vi "RvsTime_Tektronix_Vbias_crh.vi"() -> ()   [LabVIEW 2017]
uses:
  sub_vis/ke26xx/Public/Channel.ctl
  sub_vis/ke26xx/KE26XX.lvlib
panel:
  out "Total filename":string="C:\\THz-Data\\Vacuum_Box\\110725"
  in  "Heater Range (0: Off)":u16(ring) items=["Off", "Low (0.5W)", "Med (5W)", "High (50W)"]
  in  "Plot Options":enum32{"dI/dV vs V", "I vs V", "Temperature"}(tab)
  out "G vs V at neg times":cluster{"Y":dbl[], "Y":dbl[]}[](graph)
  out "G vs V at max. response":cluster{"Y":dbl[], "Y":dbl[]}[](graph)
  out "I vs V at neg times":cluster{"Y":dbl[], "Y":dbl[]}[](graph)
  out "I vs V at max. response":cluster{"Y":dbl[], "Y":dbl[]}[](graph)
  out "temp vs time":cluster{"Y":dbl[], "Y":dbl[]}[](graph)
  in  "Device Control":T1(tab)=enum."Record Data"
  in  "Lakeshore Input (0: A)":u16(ring)=2 items=["A", "B", "ITC5035"]
  in  "Lakeshore VISA Session":refnum<visa-resource-name>="COM1"
  in  "Log Temp":bool=TRUE
  in  "Heater Control":enum32{"Configure", "Heater", "Set Point"}(tab)
  in  "Curve Number (0)":dbl min=0.0 max=41.0 step=1.0
  in  "Sensor Type (0: Silicon Diode)":i8(ring) items=["Silicon Diode", "GaAIAS Diode", "100 Ohm Platinum/250", "100 Ohm Platinum/500", "1000 Ohm Platinum", "NTC RTD", "Thermo/25mV", "Thermo/50mV"]
  in  "Manual Output (%)":dbl min=0.0 max=100.0 step=0.001 format="%.;%.3f"
  in  "Loop (0: 1)":u16(ring) items=["1", "2"]
  out "Heater Output":dbl(slide) scale=0.0..100.0
  in  "Rate (D)":dbl min=0.0 max=1000.0 step=0.1 format="%.;%.1f"
  in  "Reset (I)":dbl min=0.0 max=1000.0 step=0.1 format="%.;%.1f"
  in  "Gain (P)":dbl min=0.0 max=1000.0 step=0.1 format="%.;%.1f"
  in  "Control Mode (0: Manual PID)":u16(ring) items=["Manual PID", "Zone", "Open Loop", "AutoTune PID", "AutoTune PI", "AutoTune P"]
  in  "Ramp Rate\n(K/min)":dbl=0.1 min=0.0 max=100.0 step=0.1 format="%.1f"
  in  "Ramping \nOn/Off (F: Off)":bool
  in  "Setpoint (K)":dbl min=0.0 max=1000.0 step=0.1 format="%.;%.1f"
  in  "Update":bool caption="Boolean"
  in  "Control Temp":bool=TRUE
  in  "Apply Bias":bool
  in  "Keithley VISA Session":refnum<visa-resource-name>
  in  "Channel (A):":T2
  in  "Limit (mA)":dbl=1.0 format="%.;%#_g"
  in  "Level (mV)":dbl=1.0 format="%.;%#_g"
  in  "Tektronix VISA Session":refnum<visa-resource-name>
  in  "Channel:":u16(ring) items=["Channel 1", "Channel 2", "Channel 3", "Channel 4"]
  in  "Read Scope":bool
  in  "Max. Bias (mV)":dbl=1.0 format="%.;%#_g"
  in  "Step Size (mV)":dbl=1.0 format="%.;%#_g"
  in  "Step Bias":bool
  out "Current Bias (mV)":dbl=1.0 format="%.;%#_g"
  out "Node":string
  in  "Stop 2":bool
  in  "Path":string="C:\\path\\to\\file"
  in  "Filename":string="filename"
  in  "Extension":string=".dat"
  in  "Comments":string="comments"
  in  "Start":bool
  in  "Number of Scans:":i32
  in  "Plot Scales":u16(ring) items=["Autoscale All", "Autoscale X", "Autoscale Y", "Manual Scale"]
  out "Current (mA):":dbl=19.983 format="%.;%.4f"
  out "Voltage (mV):":dbl=19.983 format="%.;%.4f"
  in  "Y Max.":dbl min=0.0 max=1000.0 step=0.1 format="%.;%.1f"
  in  "Y Min.":dbl min=0.0 max=1000.0 step=0.1 format="%.;%.1f"
  in  "X Max.":dbl min=0.0 max=1000.0 step=0.1 format="%.;%.1f"
  in  "X Min.":dbl min=0.0 max=1000.0 step=0.1 format="%.;%.1f"
  in  "Reset":bool
  out "Resistance (Ohms)":dbl=19.983 format="%.;%_5f"
  in  "Filename 2":string="07_YBCO_EOS_20K_outofplane_pumpon_5ps_"
  out "Temperature (K)":dbl=19.983 format="%.2f"
  in  "Stop":bool
  out "Osci Readout":cluster{"Y":dbl[], "Y":dbl[]}[](graph)
  # "Temperature Sensor"
  # "Heater Control"
  # "Source Meter"
  # "Oscilloscope"
  # "Set Filename and Path"
  # "(Only when not ramping bias.)"
  # "Written by Cassi Hunt, January 2013\n\nTemperature Control: LakeShore 331\nSourceMeter: Keithley 2635A\nOscilloscope: Tektronix 7xxx Series"
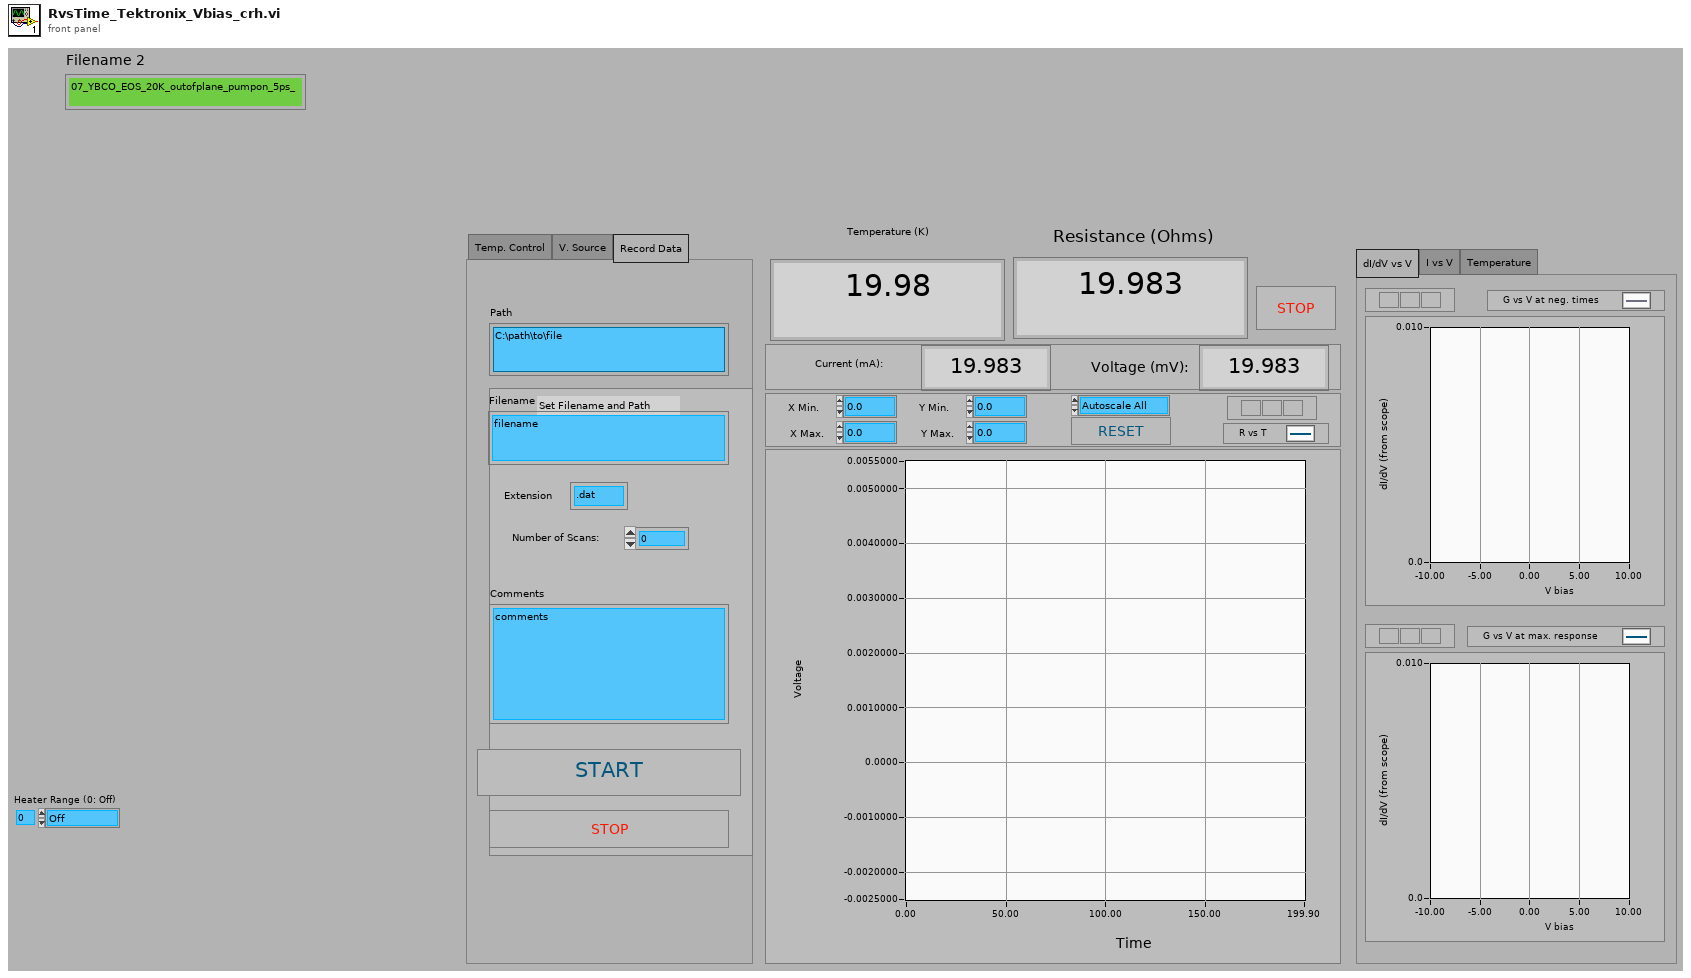
[diagram p1: front panel]
types:
  T1 = enum32{"Temp. Control", "V. Source", "Record Data"}
  T2 = typedef "KE26XX.lvlib/Channel.ctl" = enum32{"Channel A", "Channel B"}
  T3 = enum32{"Current", "Voltage", "IV", "Resistance", "Power"}
  T4 = typedef "ke26xx.lvlib/Channel.ctl" = enum32{"Channel A", "Channel B"}
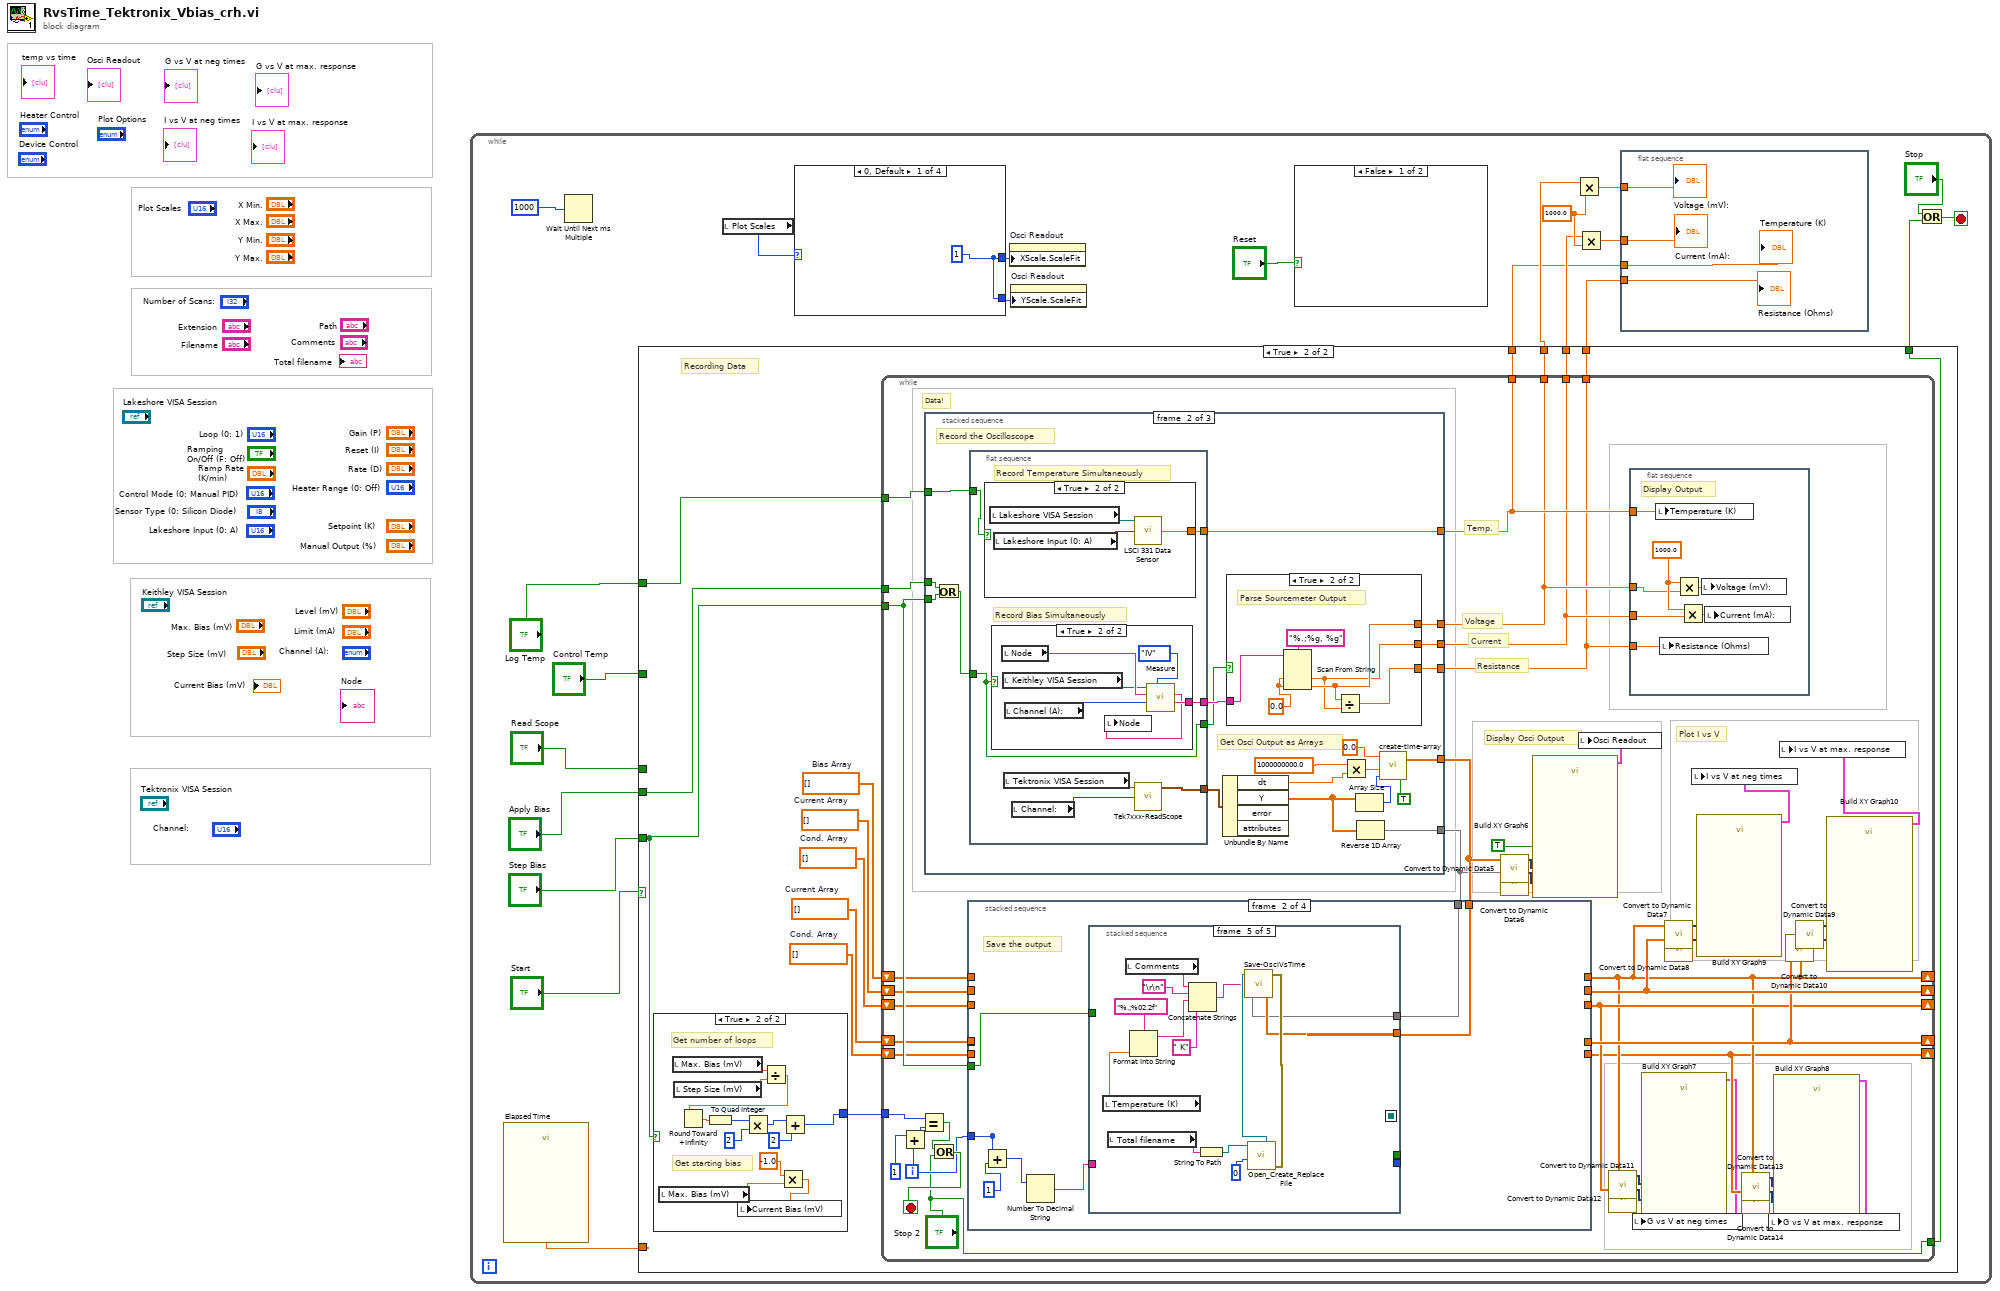
[diagram p0: block diagram]
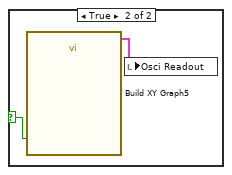
[diagram p2: hidden frame]
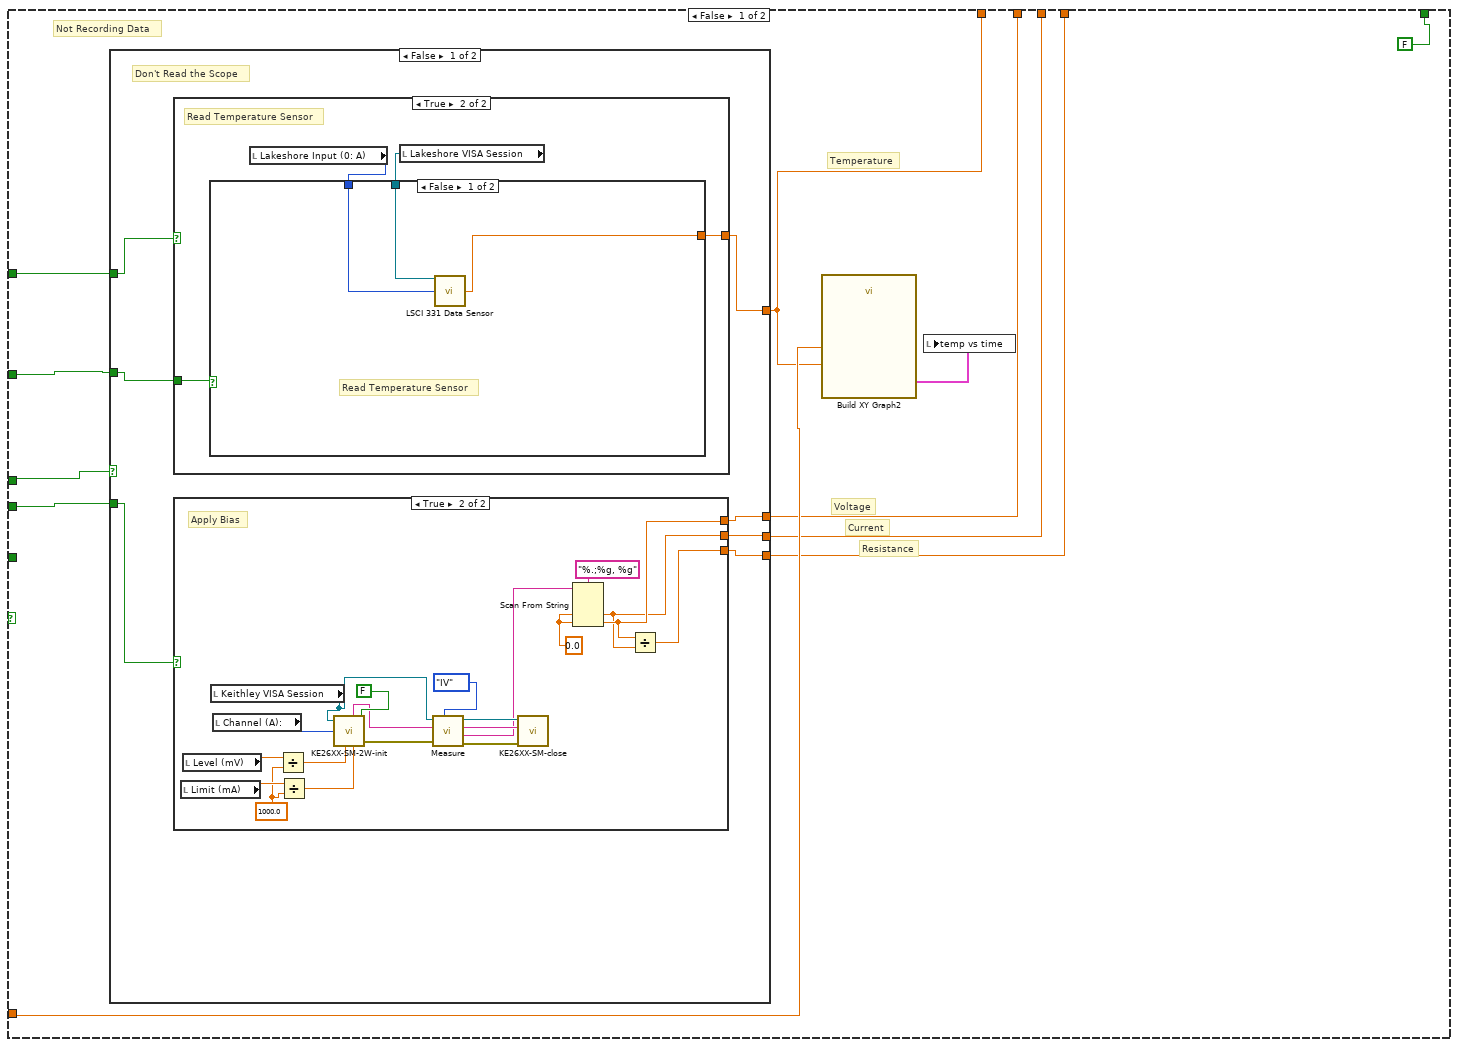
[diagram p3: hidden frame]
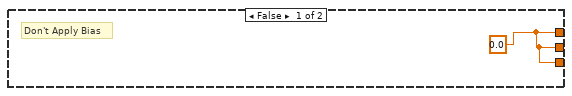
[diagram p4: hidden frame]
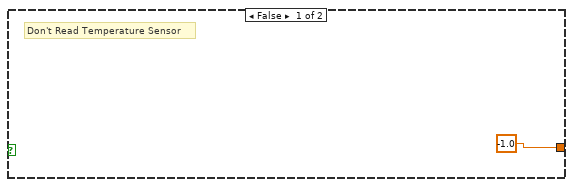
[diagram p5: hidden frame]
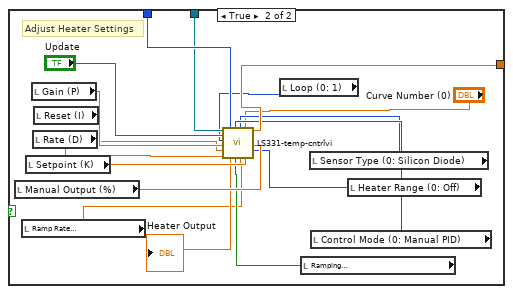
[diagram p6: hidden frame]
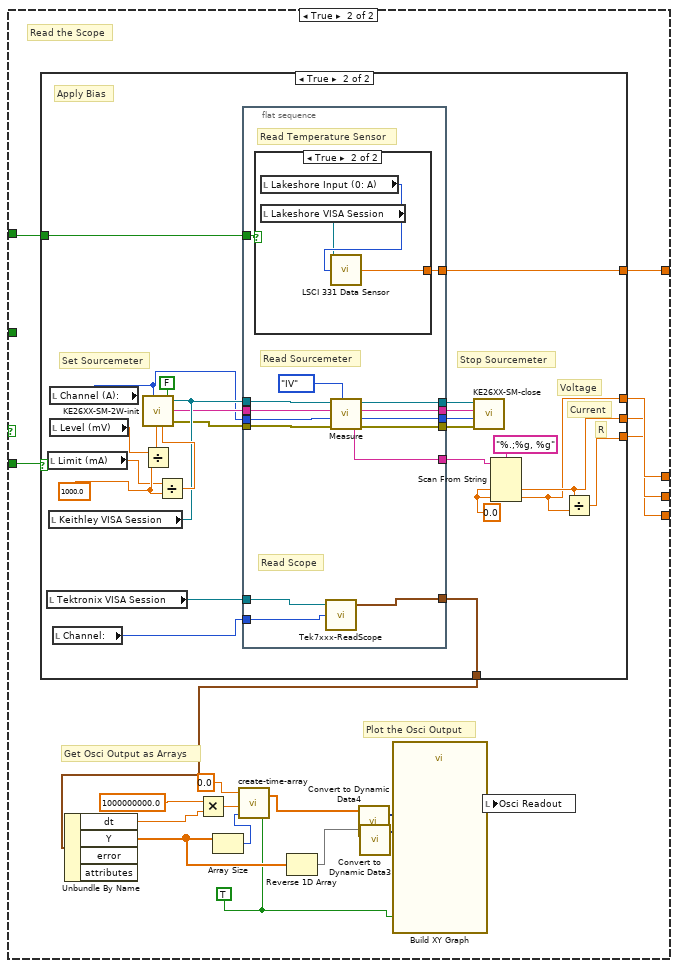
[diagram p7: hidden frame]
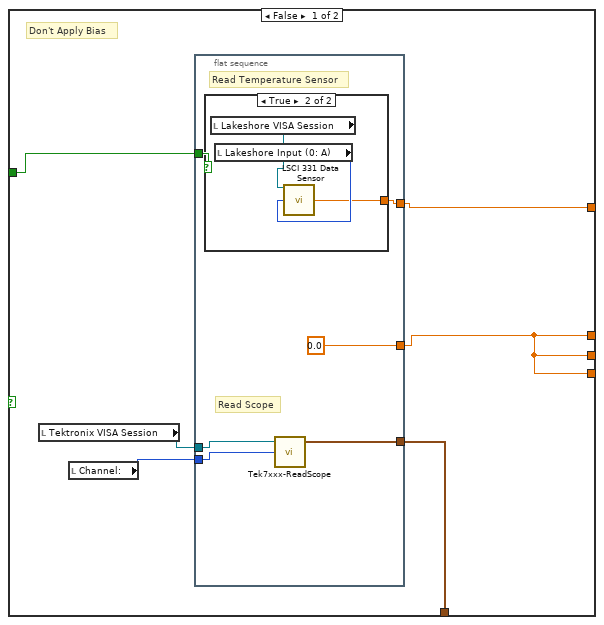
[diagram p8: hidden frame]
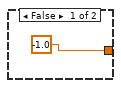
[diagram p9: hidden frame]
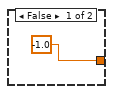
[diagram p10: hidden frame]
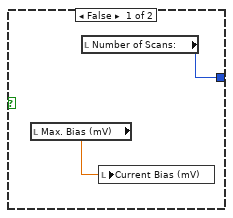
[diagram p11: hidden frame]
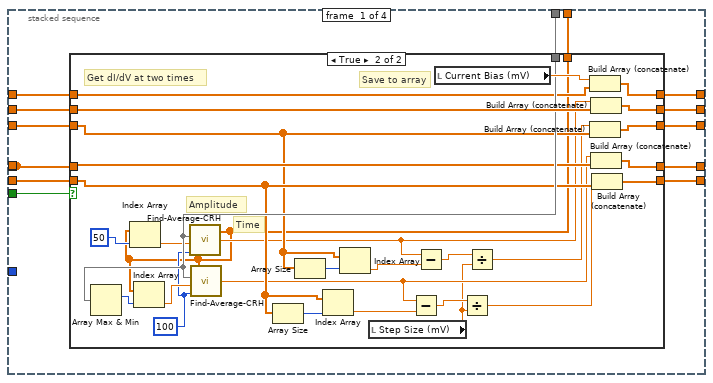
[diagram p12: hidden frame]
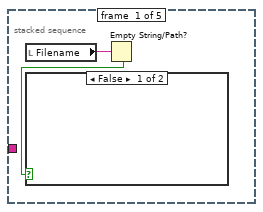
[diagram p14: hidden frame]
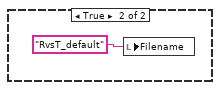
[diagram p15: hidden frame]
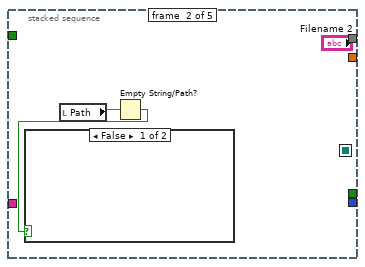
[diagram p16: hidden frame]
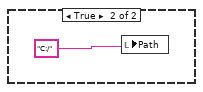
[diagram p17: hidden frame]
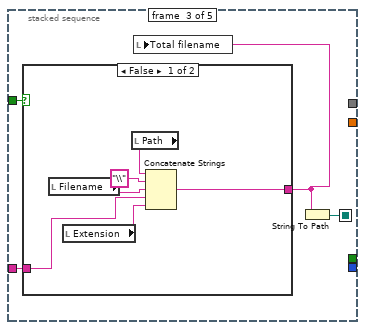
[diagram p18: hidden frame]
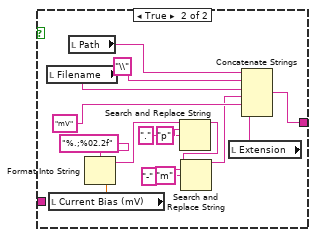
[diagram p19: hidden frame]
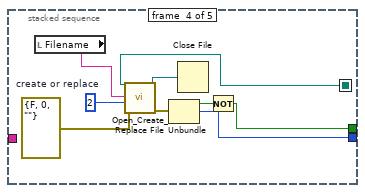
[diagram p20: hidden frame]
diagram:
  n1 = while {
    stop <- w3 stop-if-true
    w12 = 1000.0
    n2 = call "Elapsed Time"() -> ("Elapsed Time (s)"=w17:dbl)  [unwired: 12 in, 7 out]
    n3 = Wait Until Next ms Multiple(millisecond multiple=u32 1000) -> ()  [unwired: 1 out]
    n4 = case shown="True" "Start" {
      tunnel: w17 -> [w39 _]
      tunnel: "Apply Bias" -> [w35 w182]
      tunnel: [FALSE w173] -> w1
      tunnel: "Read Scope" -> [w37 _]
      tunnel: "Log Temp" -> [w36 w183]
      tunnel: "Control Temp" -> [w34 _]
      tunnel: [w33 w179] -> w9
      tunnel: [w32 w178] -> w8
      tunnel: [w31 w177] -> w7
      tunnel: [w30 w180] -> w6
      tunnel: "Step Bias" -> [_ w181]
      frame False {
        # "Temperature"
        # "Resistance"
        # "Current"
        # "Voltage"
        # "Not Recording Data"
        n5 = case shown="False" w37 {
          tunnel: w36 -> [w45 w111]
          tunnel: w35 -> [w43 w110]
          tunnel: [w44 w96] -> w30
          tunnel: w34 -> [w46 _]
          tunnel: [w42 w95] -> w33
          tunnel: [w41 w94] -> w32
          tunnel: [w40 w93] -> w31
          frame False {
            # "Don't Read the Scope"
            n6 = case shown="True" w45 {
              tunnel: [-1.0 w71] -> w44
              tunnel: w46 -> [_ w72]
              frame False {
                # "Don't Read Temperature Sensor"
              }
              frame True {
                # "Read Temperature Sensor"
                n7 = local read "Lakeshore Input (0: A)"() -> (w69:u16)
                n8 = local read "Lakeshore VISA Session"() -> (w70:refnum<visa-resource-name>)
                n9 = case shown="False" w72 {
                  tunnel: w69 -> [w74 w92]
                  tunnel: w70 -> [w75 w91]
                  tunnel: [w73 w83] -> w71
                  frame False {
                    # "Read Temperature Sensor"
                    n10 = call "LSCI 331 Data Sensor.vi"("VISA session"=w75, "Input (0: A)"=w74) -> ("Kelvin Reading"=w73:dbl)  [unwired: 1 in, 12 out]
                  }
                  frame True {
                    # "Adjust Heater Settings"
                    n11 = local read "Manual Output (%)"() -> (w85:dbl)
                    n12 = local read "Ramp Rate\n(K/min)"() -> (w80:dbl)
                    n13 = local read "Setpoint (K)"() -> (w86:dbl)
                    n14 = local read "Gain (P)"() -> (w89:dbl)
                    n15 = local read "Rate (D)"() -> (w87:dbl)
                    n16 = local read "Reset (I)"() -> (w88:dbl)
                    n17 = local read "Loop (0: 1)"() -> (w81:u16)
                    n18 = local read "Ramping \nOn/Off (F: Off)"() -> (w82:bool)
                    n19 = local read "Sensor Type (0: Silicon Diode)"() -> (w77:i8)
                    n20 = local read "Control Mode (0: Manual PID)"() -> (w78:u16)
                    n21 = local read "Heater Range (0: Off)"() -> (w79:u16)
                    n22 = call "LS331-temp-cntrlvi.vi"("VISA resource name"=w91, "Configure (False)"="Update", "Loop (0: 1)"=w81, "Gain (P) (0.0)"=w89, "Reset (I) (0.0)"=w88, "Rate (D) (0)"=w87, "Input (0: A)"=w92, "Control Mode (0: Manual PID)"=w78, "Ramping On/Off (F: Off)"=w82, "Sensor Type (0: Silicon Diode)"=w77, "Rate Value (0.1)"=w80, "Curve Number (0)"="Curve Number (0)", "Setpoint (0.0000)"=w86, "Manual Output (0.000)"=w85, "Heater Range (0: Off)"=w79) -> ("Loop 1\nHeater Output"=→"Heater Output":dbl, "Kelvin Reading"=w83:dbl)  [unwired: 1 in, 2 out]
                  }
                }
              }
            }
            n23 = case shown="True" w43 {
              tunnel: [w47 w49] -> w42
              tunnel: [w47 w48] -> w41
              tunnel: [w47 w51] -> w40
              frame False {
                w47 = 0.0
                # "Don't Apply Bias"
              }
              frame True {
                w53 = 0.0
                w63 = 1000.0
                # "Apply Bias"
                n24 = local read "Limit (mA)"() -> (w65:dbl)
                n25 = local read "Level (mV)"() -> (w67:dbl)
                n26 = local read "Keithley VISA Session"() -> (w59:refnum<visa-resource-name>)
                n27 = local read "Channel (A):"() -> (w62:T4)
                n28 = Divide(x=w67, y=w63) -> (x/y=w66:dbl)
                n29 = Divide(x=w65, y=w63) -> (x/y=w64:dbl)
                n30 = call "KE26XX-SM-2W-init.vi"("VISA resource name"=w59, "Channel (Channel A)"=w62, "Level"=w66, "Error Query (False)"=FALSE, "Limit"=w64) -> ("Node Out"=w60:string, "error out"=w58:errorcluster)  [unwired: 3 in]
                n31 = call "Measure.vi"("Function (Current)"=T3."IV" ("Measure Function (Current)"), "error in (no error)"=w58, "Node In"=w60, "VISA resource name"=w59) -> ("error out"=w54:errorcluster, "Output"=w50:string, "Node Out"=w56:string, "VISA resource name out"=w55:refnum<visa-resource-name>)  [unwired: 3 in, 1 out]
                n32 = call "KE26XX-SM-close.vi"("error in (no error)"=w54, "Node In"=w56, "VISA resource name"=w55) -> ()  [unwired: 8 in, 1 out]
                n33 = Scan From String(format string="%.;%g, %g", input string=w50, default 1=w53, default 2=w53) -> (output 1=w48:dbl, output 2=w49:dbl)  [unwired: 2 in, 3 out]
                n34 = Divide(x=w49, y=w48) -> (x/y=w51:dbl)
              }
            }
          }
          frame True {
            w100 = TRUE
            # "Plot the Osci Output"
            # "Get Osci Output as Arrays"
            # "Read the Scope"
            n35 = case shown="True" w110 {
              tunnel: w111 -> [w117 w152]
              tunnel: [w115 w128] -> w95
              tunnel: [w115 w129] -> w94
              tunnel: [w115 w134] -> w93
              tunnel: [w116 w131] -> w96
              tunnel: [w112 w130] -> w99
              frame False {
                # "Don't Apply Bias"
                n36 = local read "Tektronix VISA Session"() -> (w114:refnum<visa-resource-name>)
                n37 = local read "Channel:"() -> (w113:u16)
                n38 = flat-sequence {
                  tunnel: w117 -> [w123]
                  tunnel: [w122] -> w116
                  tunnel: [0.0] -> w115
                  tunnel: w114 -> [w120]
                  tunnel: w113 -> [w119]
                  tunnel: [w118] -> w112
                  frame #0 {
                    # "Read Scope"
                    # "Read Temperature Sensor"
                    n39 = case shown="True" w123 {
                      tunnel: [-1.0 w125] -> w122
                      frame False {
                      }
                      frame True {
                        n40 = local read "Lakeshore VISA Session"() -> (w127:refnum<visa-resource-name>)
                        n41 = local read "Lakeshore Input (0: A)"() -> (w126:u16)
                        n42 = call "LSCI 331 Data Sensor.vi"("VISA session"=w127, "Input (0: A)"=w126) -> ("Kelvin Reading"=w125:dbl)  [unwired: 1 in, 12 out]
                      }
                    }
                    n43 = call "Tek7xxx-ReadScope.vi"("Channel (0: Channel 1)"=w119, "VISA Resource Name"=w120) -> ("Waveform Graph"=w118:waveform(dbl))  [unwired: 3 in]
                  }
                }
              }
              frame True {
                w137 = 0.0
                w151 = 1000.0
                # "R"
                # "Current"
                # "Voltage"
                # "Stop Sourcemeter"
                # "Set Sourcemeter"
                # "Apply Bias"
                n44 = local read "Tektronix VISA Session"() -> (w133:refnum<visa-resource-name>)
                n45 = local read "Limit (mA)"() -> (w148:dbl)
                n46 = local read "Keithley VISA Session"() -> (w145:refnum<visa-resource-name>)
                n47 = local read "Channel (A):"() -> (w142:T4)
                n48 = local read "Level (mV)"() -> (w147:dbl)
                n49 = local read "Channel:"() -> (w132:u16)
                n50 = Divide(x=w147, y=w151) -> (x/y=w149:dbl)
                n51 = Divide(x=w148, y=w151) -> (x/y=w150:dbl)
                n52 = call "KE26XX-SM-2W-init.vi"("VISA resource name"=w145, "Channel (Channel A)"=w142, "Level"=w149, "Error Query (False)"=FALSE, "Limit"=w150) -> ("Node Out"=w144:string, "error out"=w143:errorcluster)  [unwired: 3 in]
                n53 = flat-sequence {
                  tunnel: [w166] -> w131
                  tunnel: w152 -> [w165]
                  tunnel: w144 -> [w164]
                  tunnel: w145 -> [w163]
                  tunnel: w143 -> [w162]
                  tunnel: w142 -> [w157]
                  tunnel: [w161] -> w139
                  tunnel: [w160] -> w135
                  tunnel: [w159] -> w140
                  tunnel: [w158] -> w141
                  tunnel: [w157] -> w138
                  tunnel: w133 -> [w156]
                  tunnel: w132 -> [w155]
                  tunnel: [w154] -> w130
                  frame #0 {
                    # "Read Scope"
                    # "Read Sourcemeter"
                    # "Read Temperature Sensor"
                    n54 = case shown="True" w165 {
                      tunnel: [-1.0 w168] -> w166
                      frame False {
                      }
                      frame True {
                        n55 = local read "Lakeshore Input (0: A)"() -> (w170:u16)
                        n56 = local read "Lakeshore VISA Session"() -> (w169:refnum<visa-resource-name>)
                        n57 = call "LSCI 331 Data Sensor.vi"("VISA session"=w169, "Input (0: A)"=w170) -> ("Kelvin Reading"=w168:dbl)  [unwired: 1 in, 12 out]
                      }
                    }
                    n58 = call "Tek7xxx-ReadScope.vi"("Channel (0: Channel 1)"=w155, "VISA Resource Name"=w156) -> ("Waveform Graph"=w154:waveform(dbl))  [unwired: 3 in]
                    n59 = call "Measure.vi"("Function (Current)"=T3."IV" ("Measure Function (Current)"), "error in (no error)"=w162, "Channel (Channel A)"=w157, "Node In"=w164, "VISA resource name"=w163) -> ("error out"=w161:errorcluster, "Output"=w160:string, "Node Out"=w159:string, "VISA resource name out"=w158:refnum<visa-resource-name>)  [unwired: 2 in, 1 out]
                  }
                }
                n60 = call "KE26XX-SM-close.vi"("error in (no error)"=w139, "Channel (Channel A)"=w138, "Node In"=w140, "VISA resource name"=w141) -> ()  [unwired: 7 in, 1 out]
                n61 = Scan From String(format string="%.;%g, %g", input string=w135, default 1=w137, default 2=w137) -> (output 1=w129:dbl, output 2=w128:dbl)  [unwired: 2 in, 3 out]
                n62 = Divide(x=w129, y=w128) -> (x/y=w134:dbl)
              }
            }
            n63 = Unbundle By Name(w99) -> ("dt"=w105:dbl, "Y"=w104:dbl[])  [unwired: 2 out]
            n64 = Multiply(x=1000000000.0, y=w105) -> (x*y=w107:dbl)
            n65 = Array Size(array=w104) -> (size(s)=w109:i32)
            n66 = call "create-time-array.vi"("Invert"=w100, "Array Size"=w109, "dt"=w107, "t0"=0.0) -> ("Time Array"=w98:dbl[])
            n67 = Reverse 1D Array(array=w104) -> (reversed array=w97:dbl[])
            n68 = call "Convert to Dynamic Data4"("Array"=w98) -> ("Dynamic Data Type"=w103:dynamicdata)  [unwired: 3 in]
            n69 = call "Convert to Dynamic Data3"("Array"=w97) -> ("Dynamic Data Type"=w102:dynamicdata)  [unwired: 3 in]
            n70 = call "Build XY Graph"("Reset"=w100, "Y Input"=w102, "X Input"=w103) -> ("XY Graph"=w101:cluster{"Y":dbl[], "Y":dbl[]}[])  [unwired: 2 in, 6 out]
            n71 = local write "Osci Readout"(w101) -> ()
          }
        }
        n72 = call "Build XY Graph2"("Y Input"=w30, "X Input"=w39) -> ("XY Graph"=w38:cluster{"Y":dbl[], "Y":dbl[]}[])  [unwired: 3 in, 6 out]
        n73 = local write "temp vs time"(w38) -> ()
      }
      frame True {
        w171 = dbl[] []  # Cond. Array
        w172 = dbl[] []  # Current Array
        w174 = dbl[] []  # Cond. Array
        w175 = dbl[] []  # Current Array
        w176 = dbl[] []  # Bias Array
        # "Recording Data"
        n74 = case shown="True" w181 {
          tunnel: [w185 w190] -> w184
          frame False {
            n75 = local read "Max. Bias (mV)"() -> (w186:dbl)
            n76 = local read "Number of Scans:"() -> (w185:i32)
            n77 = local write "Current Bias (mV)"(w186) -> ()
          }
          frame True {
            # "Get starting bias"
            # "Get number of loops"
            n78 = local read "Max. Bias (mV)"() -> (w188:dbl)
            n79 = local read "Max. Bias (mV)"() -> (w198:dbl)
            n80 = local read "Step Size (mV)"() -> (w197:dbl)
            n81 = Divide(x=w198, y=w197) -> (x/y=w196:dbl)
            n82 = Round Toward +Infinity(x=w196) -> (ceil(x): smallest int >= x=w193:dbl)
            n83 = To Quad Integer(1:w193) -> (0:w192:i64)
            n84 = Multiply(x=w192, y=2) -> (x*y=w194:i64)
            n85 = Multiply(x=-1.0, y=w188) -> (x*y=w187:dbl)
            n86 = local write "Current Bias (mV)"(w187) -> ()
            n87 = Add(x=w194, y=2) -> (x+y=w190:i64)
          }
        }
        n88 = while {
          tunnel: w184 -> [w240]
          tunnel: w183 -> [w239]
          tunnel: w182 -> [w238]
          tunnel: w181 -> [w227]
          tunnel: [w237] -> w180
          tunnel: [w236] -> w179
          tunnel: [w235] -> w178
          tunnel: [w234] -> w177
          shift-right: [w210] -> _
          shift-left: w176 -> [w226]
          shift-right: [w218] -> _
          shift-left: w175 -> [w225]
          shift-right: [w212] -> _
          shift-left: w174 -> [w224]
          tunnel: ["Stop 2"] -> w173
          shift-right: [w215] -> _
          shift-left: w172 -> [w221]
          shift-right: [w208] -> _
          shift-left: w171 -> [w220]
          i -> [w202]
          stop <- w222 stop-if-true
          # "Plot I vs V"
          # "Display Osci Output"
          # "Resistance"
          # "Current"
          # "Voltage"
          # "Temp."
          # "Data!"
          n89 = Add(x=1, y=w202) -> (x+y=w200:i32)
          n90 = Equal?(x=w240, y=w200) -> (x = y?=w223:bool)
          n91 = stacked-sequence {
            tunnel: w239 -> [_ w389 _]
            tunnel: [_ w388 _] -> w237
            tunnel: w238 -> [w367 w385 w424]
            tunnel: w227 -> [w366 w384 w422]
            tunnel: [_ w387 _] -> w228
            tunnel: [_ w386 _] -> w229
            tunnel: [_ w380 _] -> w236
            tunnel: [_ w379 _] -> w235
            tunnel: [_ w378 _] -> w234
            frame #0 {
              n92 = Or(x=w367, y=w366) -> (x .or. y?=w368:bool)
              n93 = case shown="True" w368 {
                frame False {
                }
                frame True {
                  w375 = 1000.0
                  # "Apply Bias"
                  n94 = local read "Keithley VISA Session"() -> (w371:refnum<visa-resource-name>)
                  n95 = local read "Current Bias (mV)"() -> (w377:dbl)
                  n96 = local read "Channel (A):"() -> (w370:T4)
                  n97 = local read "Limit (mA)"() -> (w376:dbl)
                  n98 = Divide(x=w377, y=w375) -> (x/y=w374:dbl)
                  n99 = Divide(x=w376, y=w375) -> (x/y=w373:dbl)
                  n100 = call "KE26XX-SM-2W-init.vi"("VISA resource name"=w371, "Channel (Channel A)"=w370, "Level"=w374, "Error Query (False)"=FALSE, "Limit"=w373) -> ("Node Out"=w369:string)  [unwired: 3 in, 1 out]
                  n101 = local write "Node"(w369) -> ()
                }
              }
            }
            frame #1 {
              # "Get Osci Output as Arrays"
              # "Record the Oscilloscope"
              n102 = Or(x=w385, y=w384) -> (x .or. y?=w383:bool)
              n103 = flat-sequence {
                tunnel: w389 -> [w411]
                tunnel: [w410] -> w388
                tunnel: [w407] -> w397
                tunnel: w383 -> [w405]
                tunnel: [w406] -> w382
                tunnel: [w405] -> w381
                frame #0 {
                  # "Record Bias Simultaneously"
                  # "Record Temperature Simultaneously"
                  n104 = case shown="True" w411 {
                    tunnel: [-1.0 w419] -> w410
                    frame False {
                    }
                    frame True {
                      n105 = local read "Lakeshore VISA Session"() -> (w421:refnum<visa-resource-name>)
                      n106 = local read "Lakeshore Input (0: A)"() -> (w420:u16)
                      n107 = call "LSCI 331 Data Sensor.vi"("VISA session"=w421, "Input (0: A)"=w420) -> ("Kelvin Reading"=w419:dbl)  [unwired: 1 in, 12 out]
                    }
                  }
                  n108 = case shown="True" w405 {
                    tunnel: [_ w413] -> w406
                    frame False {
                    }
                    frame True {
                      n109 = local read "Node"() -> (w416:string)
                      n110 = local read "Keithley VISA Session"() -> (w415:refnum<visa-resource-name>)
                      n111 = local read "Channel (A):"() -> (w414:T4)
                      n112 = call "Measure.vi"("Function (Current)"=T3."IV" ("Measure Function (Current)"), "Channel (Channel A)"=w414, "Node In"=w416, "VISA resource name"=w415) -> ("Output"=w413:string, "Node Out"=w412:string)  [unwired: 3 in, 3 out]
                      n113 = local write "Node"(w412) -> ()
                    }
                  }
                  n114 = local read "Tektronix VISA Session"() -> (w409:refnum<visa-resource-name>)
                  n115 = local read "Channel:"() -> (w408:u16)
                  n116 = call "Tek7xxx-ReadScope.vi"("Channel (0: Channel 1)"=w408, "VISA Resource Name"=w409) -> ("Waveform Graph"=w407:waveform(dbl))  [unwired: 3 in]
                }
              }
              n117 = Unbundle By Name(w397) -> ("dt"=w394:dbl, "Y"=w395:dbl[])  [unwired: 2 out]
              n118 = case shown="True" w381 {
                tunnel: w382 -> [_ w402]
                tunnel: [w398 w400] -> w380
                tunnel: [w398 w399] -> w379
                tunnel: [w398 w403] -> w378
                frame False {
                  w398 = 0.0
                }
                frame True {
                  w401 = 0.0
                  # "Parse Sourcemeter Output"
                  n119 = Scan From String(format string="%.;%g, %g", input string=w402, default 1=w401, default 2=w401) -> (output 1=w399:dbl, output 2=w400:dbl)  [unwired: 2 in, 3 out]
                  n120 = Divide(x=w400, y=w399) -> (x/y=w403:dbl)
                }
              }
              n121 = Multiply(x=1000000000.0, y=w394) -> (x*y=w392:dbl)
              n122 = Array Size(array=w395) -> (size(s)=w390:i32)
              n123 = Reverse 1D Array(array=w395) -> (reversed array=w387:dbl[])
              n124 = call "create-time-array.vi"("Invert"=TRUE, "Array Size"=w390, "dt"=w392, "t0"=0.0) -> ("Time Array"=w386:dbl[])
            }
            frame #2 {
              n125 = Or(x=w424, y=w422) -> (x .or. y?=w423:bool)
              n126 = case shown="True" w423 {
                frame False {
                }
                frame True {
                  # "Stop Sourcemeter"
                  n127 = local read "Keithley VISA Session"() -> (w427:refnum<visa-resource-name>)
                  n128 = local read "Channel (A):"() -> (w425:T4)
                  n129 = local read "Node"() -> (w426:string)
                  n130 = call "KE26XX-SM-close.vi"("Channel (Channel A)"=w425, "Node In"=w426, "VISA resource name"=w427) -> ()  [unwired: 8 in, 1 out]
                }
              }
            }
          }
          n131 = Or(x=w223, y="Stop 2") -> (x .or. y?=w222:bool)
          n132 = stacked-sequence {
            tunnel: w229 -> [w251 w289 _ _]
            tunnel: w228 -> [w252 w290 _ _]
            tunnel: w227 -> [w253 w288 w349 _]
            tunnel: w226 -> [w250 _ _ _]
            tunnel: w225 -> [w249 _ _ _]
            tunnel: w224 -> [w248 _ _ _]
            tunnel: [w247 _ _ _] -> w210
            tunnel: [w246 _ _ _] -> w218
            tunnel: [w245 _ _ _] -> w212
            tunnel: [w244 _ _ _] -> _
            tunnel: w221 -> [w244 _ _ _]
            tunnel: [w243 _ _ _] -> w215
            tunnel: w220 -> [w242 _ _ _]
            tunnel: [w241 _ _ _] -> w208
            tunnel: [_ w293 _ _] -> _
            tunnel: w202 -> [_ w293 _ _]
            frame #0 {
              n133 = case shown="True" w253 {
                tunnel: w252 -> [_ w282]
                tunnel: w251 -> [_ w259]
                tunnel: w250 -> [w258 w262]
                tunnel: w249 -> [w257 w287]
                tunnel: w248 -> [w256 w272]
                tunnel: [w258 w286] -> w247
                tunnel: [w257 w285] -> w246
                tunnel: [w256 w284] -> w245
                tunnel: w244 -> [w255 w278]
                tunnel: [w255 w277] -> w243
                tunnel: [w254 w276] -> w241
                tunnel: w242 -> [w254 w273]
                frame False {
                }
                frame True {
                  w279 = 100
                  # "Time"
                  # "Amplitude"
                  # "Save to array"
                  # "Get dI/dV at two times"
                  n134 = Array Max & Min(array=w282) -> (max index (indices)=w281:i32)  [unwired: 3 out]
                  n135 = Index Array(array=w259, index=50) -> (element=w260:dbl)
                  n136 = Index Array(array=w259, index=w281) -> (element=w280:dbl)
                  n137 = call "Find-Average-CRH.vi"("Number to average"=w279, "t0"=w260, "Amplitude Array"=w282, "Time Array"=w259) -> ("Averaged Amplitude"=w271:dbl)
                  n138 = call "Find-Average-CRH.vi"("Number to average"=w279, "t0"=w280, "Amplitude Array"=w282, "Time Array"=w259) -> ("Averaged Amplitude"=w268:dbl)
                  n139 = Array Size(array=w273) -> (size(s)=w274:i32)
                  n140 = Array Size(array=w272) -> (size(s)=w275:i32)
                  n141 = Index Array(array=w273, index=w274) -> (element=w267:dbl)
                  n142 = Index Array(array=w272, index=w275) -> (element=w270:dbl)
                  n143 = local read "Step Size (mV)"() -> (w265:dbl)
                  n144 = Subtract(x=w268, y=w267) -> (x-y=w266:dbl)
                  n145 = Subtract(x=w271, y=w270) -> (x-y=w269:dbl)
                  n146 = local read "Current Bias (mV)"() -> (w283:dbl)
                  n147 = Divide(x=w266, y=w265) -> (x/y=w263:dbl)
                  n148 = Divide(x=w269, y=w265) -> (x/y=w264:dbl)
                  n149 = Build Array (concatenate)(w283, w262) -> (w286:dbl[])
                  n150 = Build Array (concatenate)(w264, w272) -> (w284:dbl[])
                  n151 = Build Array (concatenate)(w271, w287) -> (w285:dbl[])
                  n152 = Build Array (concatenate)(w268, w278) -> (w277:dbl[])
                  n153 = Build Array (concatenate)(w263, w273) -> (w276:dbl[])
                }
              }
            }
            frame #1 {
              # "Save the output"
              n154 = Add(x=w293, y=1) -> (x+y=w294:i32)
              n155 = Number To Decimal String(number=w294) -> (decimal integer string=w291:string)  [unwired: 1 in]
              n156 = stacked-sequence {
                seq-local: [_ _ w304 _ _] -> [_ _ _ w328 _]
                tunnel: [_ _ _ w329 _] -> _
                tunnel: [_ _ _ w327 _] -> _
                tunnel: w291 -> [_ _ w303 _ _]
                tunnel: w289 -> [_ _ _ _ w340]
                tunnel: w290 -> [_ _ _ _ w339]
                tunnel: w288 -> [_ _ w301 _ _]
                frame #0 {
                  n157 = local read "Filename"() -> (w296:string)
                  n158 = Empty String/Path?(string/path=w296) -> (empty?=w295:bool)
                  n159 = case shown="False" w295 {
                    frame False {
                    }
                    frame True {
                      n160 = local write "Filename"("RvsT_default") -> ()
                    }
                  }
                }
                frame #1 {
                  n161 = local read "Path"() -> (w299:string)
                  n162 = Empty String/Path?(string/path=w299) -> (empty?=w298:bool)
                  n163 = case shown="False" w298 {
                    frame False {
                    }
                    frame True {
                      n164 = local write "Path"("C:/") -> ()
                    }
                  }
                }
                frame #2 {
                  n165 = case shown="False" w301 {
                    tunnel: w303 -> [w306 _]
                    tunnel: [w305 w322] -> w302
                    frame False {
                      n166 = local read "Filename"() -> (w309:string)
                      n167 = local read "Extension"() -> (w310:string)
                      n168 = local read "Path"() -> (w308:string)
                      n169 = Concatenate Strings(w308, "\\" ("Substring"), w309, w306, w310) -> (w305:string)
                    }
                    frame True {
                      n170 = local read "Filename"() -> (w323:string)
                      n171 = local read "Current Bias (mV)"() -> (w319:dbl)
                      n172 = local read "Path"() -> (w325:string)
                      n173 = Format Into String(format string="%.;%02.2f", w319) -> (resulting string=w313:string)  [unwired: 2 in, 1 out]
                      n174 = Search and Replace String(input string=w313, search string=".", replace string="p" ("replace string (\"\")")) -> (result string=w312:string)  [unwired: 5 in, 3 out]
                      n175 = Search and Replace String(input string=w312, search string="-", replace string="m" ("replace string (\"\")")) -> (result string=w311:string)  [unwired: 5 in, 3 out]
                      n176 = local read "Extension"() -> (w320:string)
                      n177 = Concatenate Strings(w325, "\\" ("Substring"), w323, w311, "mV" ("Substring"), w320) -> (w322:string)
                    }
                  }
                  n178 = local write "Total filename"(w302) -> ()
                  n179 = String To Path(string=w302) -> (path=w304:path)
                }
                frame #3 {
                  w331 = i16 2  # create or replace
                  n180 = local read "Filename"() -> (w326:string)
                  n181 = call <vilib>:"Open_Create_Replace File.vi"("default name"=w326, "error in (no error)"=errorcluster {"status"=FALSE, "code"=0, "source"=""}, "function (open:0)"=w331, "file path"=w328) -> ("error out"=w333:errorcluster, "refnum"=w332:refnum<file>)  [unwired: 2 in, 4 out]
                  n182 = Unbundle(w333) -> ("status"=w330:bool, "code"=w327:i32)  [unwired: 1 out]
                  n183 = Close File(refnum=w332) -> ()  [unwired: 1 in, 2 out]
                  n184 = Not(x=w330) -> (.not. x?=w329:bool)
                }
                frame #4 {
                  n185 = local read "Temperature (K)"() -> (w336:dbl)
                  n186 = local read "Total filename"() -> (w342:string)
                  n187 = local read "Comments"() -> (w344:string)
                  n188 = Format Into String(format string="%.;%02.2f", w336) -> (resulting string=w337:string)  [unwired: 2 in, 1 out]
                  n189 = Concatenate Strings(w344, "\r\n", w337, " K" ("format string")) -> (w345:string)
                  n190 = String To Path(string=w342) -> (path=w341:path)
                  n191 = call <vilib>:"Open_Create_Replace File.vi"("function (open:0)"=i16 0 ("create or replace"), "file path"=w341) -> ("error out"=w347:errorcluster, "refnum"=w348:refnum<file>)  [unwired: 4 in, 4 out]
                  n192 = call "Save-OsciVsTime.vi"("X-Values"=w340, "error in"=w347, "Y-Values"=w339, "comment"=w345, "refnum"=w348) -> ()  [unwired: 1 out]
                }
              }
            }
            frame #2 {
              n193 = case shown="True" w349 {
                frame False {
                }
                frame True {
                  # "Step Bias"
                  n194 = local read "Current Bias (mV)"() -> (w355:dbl)
                  n195 = local read "Step Size (mV)"() -> (w354:dbl)
                  n196 = local read "Max. Bias (mV)"() -> (w351:dbl)
                  n197 = Add(x=w355, y=w354) -> (x+y=w352:dbl)
                  n198 = Greater?(x=w352, y=w351) -> (0:w353:bool)
                  n199 = case shown="False" w353 {
                    tunnel: w352 -> [w356 _]
                    tunnel: w351 -> [_ w357]
                    tunnel: [w356 w357] -> w350
                    frame False {
                    }
                    frame True {
                    }
                  }
                  n200 = local write "Current Bias (mV)"(w350) -> ()
                }
              }
            }
            frame #3 {
              # "Wait"
              n201 = Wait (ms)(milliseconds to wait=300) -> ()  [unwired: 1 out]
            }
          }
          n202 = call "Convert to Dynamic Data5"("Array"=w229) -> ("Dynamic Data Type"=w233:dynamicdata)  [unwired: 3 in]
          n203 = call "Convert to Dynamic Data6"("Array"=w228) -> ("Dynamic Data Type"=w232:dynamicdata)  [unwired: 3 in]
          n204 = call "Build XY Graph6"("Reset"=TRUE, "Y Input"=w232, "X Input"=w233) -> ("XY Graph"=w230:cluster{"Y":dbl[], "Y":dbl[]}[])  [unwired: 2 in, 6 out]
          n205 = local write "Osci Readout"(w230) -> ()
          n206 = call "Convert to Dynamic Data11"("Array"=w210) -> ("Dynamic Data Type"=w213:dynamicdata)  [unwired: 3 in]
          n207 = call "Convert to Dynamic Data12"("Array"=w212) -> ("Dynamic Data Type"=w211:dynamicdata)  [unwired: 3 in]
          n208 = flat-sequence {
            tunnel: w237 -> [w365]
            tunnel: w236 -> [w362]
            tunnel: w235 -> [w361]
            tunnel: w234 -> [w364]
            frame #0 {
              w363 = 1000.0
              # "Display Output"
              n209 = local write "Temperature (K)"(w365) -> ()
              n210 = local write "Resistance (Ohms)"(w364) -> ()
              n211 = Multiply(x=w363, y=w362) -> (x*y=w360:dbl)
              n212 = Multiply(x=w363, y=w361) -> (x*y=w359:dbl)
              n213 = local write "Voltage (mV):"(w360) -> ()
              n214 = local write "Current (mA):"(w359) -> ()
            }
          }
          n215 = call "Build XY Graph7"("Y Input"=w211, "X Input"=w213) -> ("XY Graph"=w204:cluster{"Y":dbl[], "Y":dbl[]}[])  [unwired: 3 in, 6 out]
          n216 = local write "G vs V at neg times"(w204) -> ()
          n217 = call "Convert to Dynamic Data7"("Array"=w210) -> ("Dynamic Data Type"=w219:dynamicdata)  [unwired: 3 in]
          n218 = call "Convert to Dynamic Data8"("Array"=w218) -> ("Dynamic Data Type"=w217:dynamicdata)  [unwired: 3 in]
          n219 = call "Build XY Graph9"("Y Input"=w217, "X Input"=w219) -> ("XY Graph"=w206:cluster{"Y":dbl[], "Y":dbl[]}[])  [unwired: 3 in, 6 out]
          n220 = local write "I vs V at neg times"(w206) -> ()
          n221 = call "Convert to Dynamic Data13"("Array"=w210) -> ("Dynamic Data Type"=w209:dynamicdata)  [unwired: 3 in]
          n222 = call "Convert to Dynamic Data14"("Array"=w208) -> ("Dynamic Data Type"=w207:dynamicdata)  [unwired: 3 in]
          n223 = call "Build XY Graph8"("Y Input"=w207, "X Input"=w209) -> ("XY Graph"=w203:cluster{"Y":dbl[], "Y":dbl[]}[])  [unwired: 3 in, 6 out]
          n224 = local write "G vs V at max. response"(w203) -> ()
          n225 = call "Convert to Dynamic Data10"("Array"=w215) -> ("Dynamic Data Type"=w214:dynamicdata)  [unwired: 3 in]
          n226 = call "Convert to Dynamic Data9"("Array"=w210) -> ("Dynamic Data Type"=w216:dynamicdata)  [unwired: 3 in]
          n227 = call "Build XY Graph10"("Y Input"=w214, "X Input"=w216) -> ("XY Graph"=w205:cluster{"Y":dbl[], "Y":dbl[]}[])  [unwired: 3 in, 6 out]
          n228 = local write "I vs V at max. response"(w205) -> ()
        }
      }
    }
    n229 = local read "Plot Scales"() -> (w21:u16)
    n230 = case shown="0, Default" w21 {
      tunnel: [w428 1 0 w441] -> w19
      tunnel: [w428 0 1 w441] -> w20
      frame 0, Default {
        w428 = 1
      }
      frame 1 {
        n231 = local read "Y Max."() -> (w431:dbl)
        n232 = local read "Y Min."() -> (w432:dbl)
        n233 = property on="Osci Readout" class="XYGraph (strict)"("YScale.Maximum"=w431, "YScale.Minimum"=w432) -> ()  [unwired: 2 in, 2 out]
      }
      frame 2 {
        n234 = local read "X Max."() -> (w436:dbl)
        n235 = local read "X Min."() -> (w435:dbl)
        n236 = property on="Osci Readout" class="XYGraph (strict)"("XScale.Maximum"=w436, "XScale.Minimum"=w435) -> ()  [unwired: 2 in, 2 out]
      }
      frame 3 {
        w441 = 0
        n237 = local read "X Max."() -> (w440:dbl)
        n238 = local read "X Min."() -> (w439:dbl)
        n239 = local read "Y Max."() -> (w438:dbl)
        n240 = local read "Y Min."() -> (w437:dbl)
        n241 = property on="Osci Readout" class="XYGraph (strict)"("XScale.Maximum"=w440, "XScale.Minimum"=w439) -> ()  [unwired: 2 in, 2 out]
        n242 = property on="Osci Readout" class="XYGraph (strict)"("YScale.Maximum"=w438, "YScale.Minimum"=w437) -> ()  [unwired: 2 in, 2 out]
      }
    }
    n243 = property on="Osci Readout" class="XYGraph (strict)"("XScale.ScaleFit"=w19) -> ()  [unwired: 2 in, 2 out]
    n244 = property on="Osci Readout" class="XYGraph (strict)"("YScale.ScaleFit"=w20) -> ()  [unwired: 2 in, 2 out]
    n245 = case shown="False" "Reset" {
      selector: "Reset" -> [_ w23]
      frame False {
      }
      frame True {
        n246 = call "Build XY Graph5"("Reset"=w23) -> ("XY Graph"=w24:cluster{"Y":dbl[], "Y":dbl[]}[])  [unwired: 4 in, 6 out]
        n247 = local write "Osci Readout"(w24) -> ()
      }
    }
    n248 = Multiply(x=w9, y=w12) -> (x*y=w11:dbl)
    n249 = Multiply(x=w8, y=w12) -> (x*y=w10:dbl)
    n250 = flat-sequence {
      tunnel: w11 -> [w28]
      tunnel: w10 -> [w27]
      tunnel: w7 -> [w26]
      tunnel: w6 -> [w25]
      frame #0 {
        "Voltage (mV):" <- w28
        "Current (mA):" <- w27
        "Temperature (K)" <- w25
        "Resistance (Ohms)" <- w26
      }
    }
    n251 = Or(x="Stop", y=w1) -> (x .or. y?=w3:bool)
  }
